vi "Log (SubVI).vi"(7 "Msgtype":u16(ring) items=["send", "recieved", "other"], 9 "String":string, 11 "file path (use dialog)":path) -> (3 "path":path)   [LabVIEW 2014]
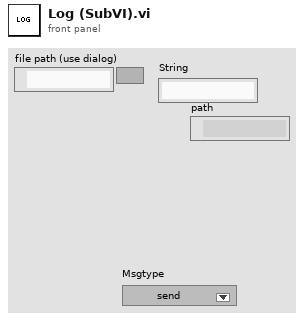
[diagram p1: front panel]
types:
  T1 = enum16{"open", "replace", "create", "open or create", "replace or create", "replace or create with confirmation"}
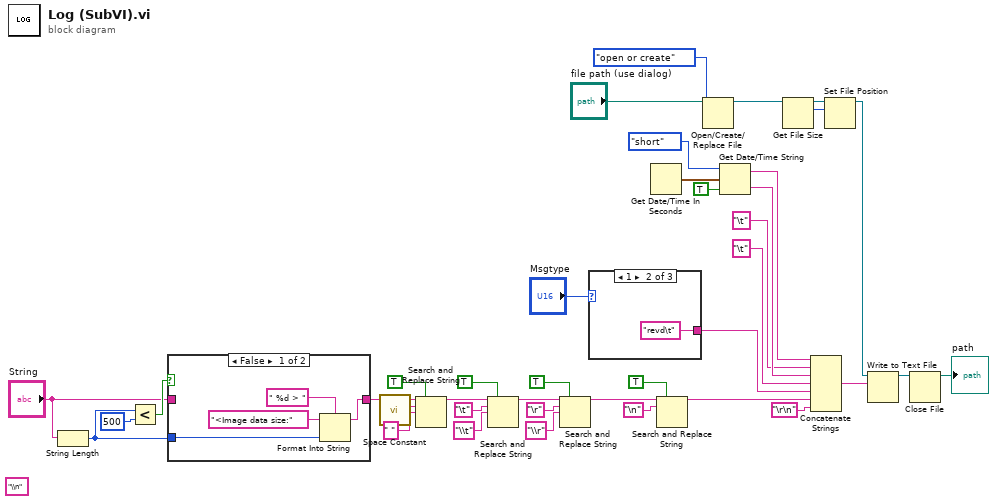
[diagram p0: block diagram]
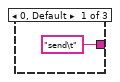
[diagram p3: hidden frame]
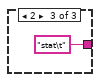
[diagram p4: hidden frame]
diagram:
  (unwired) "\\n" ("replace string (\"\")")
  n1 = String Length(string="String") -> (length=w20:i32)
  n2 = Less?(x=w20, y=500) -> (x < y?=w22:bool)
  n3 = case shown="False" w22 {
    tunnel: "String" -> [_ w44]
    tunnel: [w40 w44] -> w19
    tunnel: w20 -> [w41 _]
    frame False {
      n4 = Format Into String(format string=" %d > ", initial string="<Image data size:" ("String"), w41) -> (resulting string=w40:string)  [unwired: 1 in, 1 out]
    }
    frame True {
    }
  }
  n5 = call <vilib>:"Space Constant.vi"() -> ("String"=w16:string)
  n6 = Search and Replace String(replace all?=TRUE ("replace all? (F)"), input string=w19, search string=w16, replace string=" " ("replace string (\"\")")) -> (result string=w18:string)  [unwired: 4 in, 3 out]
  n7 = Search and Replace String(replace all?=TRUE ("replace all? (F)"), input string=w18, search string="\t", replace string="\\t" ("replace string (\"\")")) -> (result string=w17:string)  [unwired: 4 in, 3 out]
  n8 = Search and Replace String(replace all?=TRUE ("replace all? (F)"), input string=w17, search string="\r", replace string="\\r" ("replace string (\"\")")) -> (result string=w5:string)  [unwired: 4 in, 3 out]
  n9 = case shown="1" "Msgtype" {
    tunnel: ["send\t" ("string") "revd\t" ("string") "stat\t" ("string")] -> w2
    frame 0, Default {
    }
    frame 1 {
    }
    frame 2 {
    }
  }
  n10 = Get Date/Time In Seconds() -> (seconds since 1Jan1904=w33:timestamp)
  n11 = Search and Replace String(replace all?=TRUE ("replace all? (F)"), input string=w5, search string="\n") -> (result string=w4:string)  [unwired: 5 in, 3 out]
  n12 = Open/Create/Replace File(file path (use dialog)="file path (use dialog)", operation (0:open)=T1."open or create") -> (refnum out=w27:refnum<file>)  [unwired: 4 in, 2 out]
  n13 = Get Date/Time String(date format (0)=enum16{"short", "long", "abbreviated"}."short", seconds (now)=w33, want seconds? (F)=TRUE) -> (date string=w36:string, time string=w38:string)
  n14 = Get File Size(file=w27) -> (refnum out=w26:refnum<file>, size (in bytes)=w24:i64)  [unwired: 1 in, 1 out]
  n15 = Concatenate Strings(w36, "\t" ("string"), w38, "\t" ("string"), w2, w4, "\r\n") -> (w39:string)
  n16 = Set File Position(offset (in bytes) (0)=w24, refnum=w26) -> (refnum out=w25:refnum<file>)  [unwired: 2 in, 1 out]
  n17 = Write to Text File(file (use dialog)=w25, text=w39) -> (refnum out=w29:refnum<file>)  [unwired: 2 in, 2 out]
  n18 = Close File(refnum=w29) -> (path=→"path":path)  [unwired: 1 in, 1 out]
